vi "SEWV Specific Enthalpy of Water Vapor (KJ to Kg).vi"(1 "Tceg":dbl[unit]) -> (0 "SEWV":dbl[unit])   [LabVIEW 2018]
panel:
  out "Temprature Of Input Air\nKelvin Degree":dbl[unit](slide) scale=273.0..373.0
  out "Tk":dbl[unit]
  out "SEWV Specific Enthalpy of Water Vapor\nSEWV=SHCWV*Tk+LHWE;":dbl[unit](knob)
  out "Temprature Of Input Air\nCentigrade Degree":dbl[unit](slide) scale=0.0..100.0
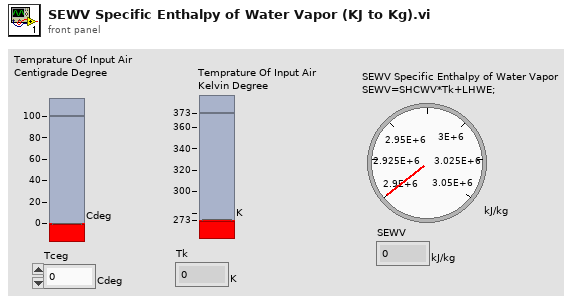
[diagram p1: front panel]
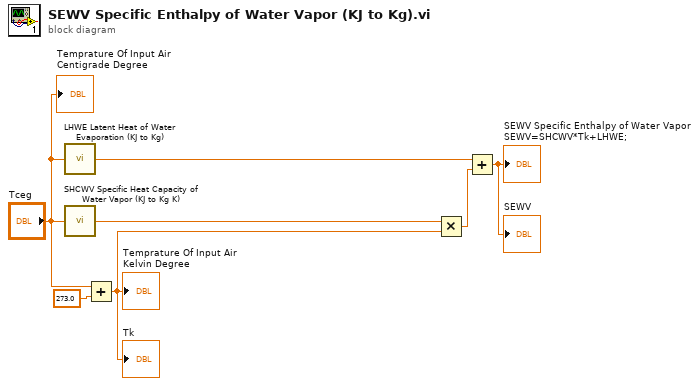
[diagram p0: block diagram]
diagram:
  n1 = call "LHWE Latent Heat of Water Evaporation (KJ to Kg).vi"("Tceg"="Tceg") -> ("LHWE"=w3:dbl[unit])
  n2 = call "SHCWV Specific Heat Capacity of Water Vapor (KJ to Kg K).vi"("Tceg"="Tceg") -> ("SHCWV"=w2:dbl[unit])
  n3 = Add(x="Tceg", y=dbl[unit] 273.0) -> (x+y=w4:dbl[unit])
  "Tk" <- w4
  "Temprature Of Input Air\nKelvin Degree" <- w4
  n4 = Multiply(x=w2, y=w4) -> (x*y=w5:dbl[unit])
  n5 = Add(x=w3, y=w5) -> (x+y=→"SEWV Specific Enthalpy of Water Vapor\nSEWV=SHCWV*Tk+LHWE;" →"SEWV":dbl[unit])
  "Temprature Of Input Air\nCentigrade Degree" <- "Tceg"
